vi "Initialize.vi"(8 "error in":errorcluster, 11 "device data model in":refnum<class "Device Data Model.lvclass">) -> (0 "error out":errorcluster, 3 "device data model out":refnum<class "Device Data Model.lvclass">)   [LabVIEW 2015, in "Modbus Library.lvlib" / "Device Data Model.lvclass"]
doc: "This VI initializes the device data model."
uses:
  Device Data Model.lvclass
  Device Data Model.lvclass/Device Data Model.ctl
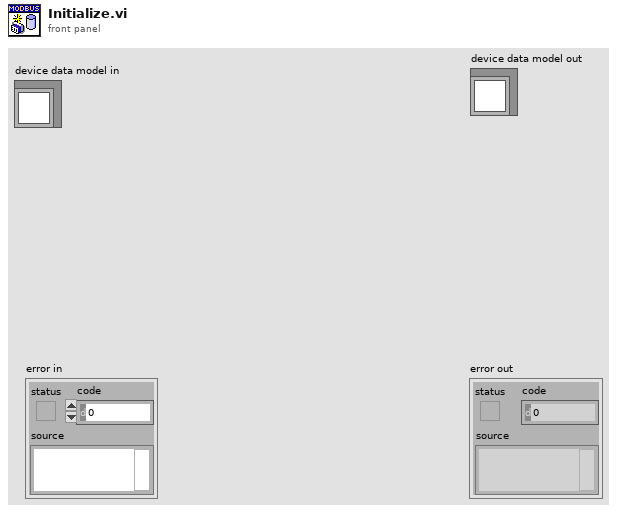
[diagram p1: front panel]
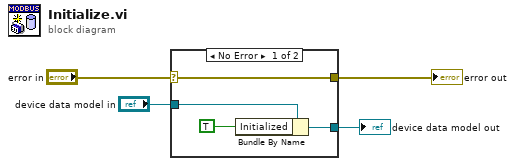
[diagram p0: block diagram]
diagram:
  n1 = case shown="No Error" "error in" {
    selector: "error in" -> [w5 w10]
    tunnel: "device data model in" -> [w8 w9]
    tunnel: [w6 w9] -> w3
    tunnel: [w5 w10] -> w1
    frame No Error {
      n2 = Bundle By Name(cluster=w8, "Initialized"=TRUE) -> (w6:refnum<class "Device Data Model.lvclass">)
    }
    frame Error {
    }
  }
  "error out" <- w1
  "device data model out" <- w3
